vi "U6 Two 32-bit Frequency Measurements.vi"() -> ()   [LabVIEW 2021]
panel:
  in  "DeviceType":u16(ring)=1 items=["LJ_dtU3", "LJ_dtU6", "LJ_dtUE9"]
  out "Counter1 Diff (FIO3)":u32
  out "Frequency (FIO1)":dbl format="%.2f"
  out "Period (FIO1)":dbl format="%.6f"
  out "Iteration":i32
  out "Frequency (FIO0)":dbl format="%.2f"
  out "Period (FIO0)":dbl format="%.6f"
  in  "error in":errorcluster
  in  "ConnectionType":u16(ring) items=["LJ_ctUSB", "LJ_ctETHERNET"]
  in  "Address":string="1"
  in  "FirstFound":bool=TRUE
  in  "stop":bool
  out "Counter0 Diff (FIO2)":u32
  out "error out":errorcluster
  out "Error Message":string
  # "Each iteration, this VI measures the frequency on FIO0 and FIO1 using timer mode 2 (32-bit\nperiod measurement).  Also reads the count on FIO2 and FIO3 and\ndisplays the difference from the previous iteration, with the idea that the same signal can\nbe connected to FIO0 and FIO2 (and to FIO1 and FIO3) for comparison of period timing\nversus pulse counting."
  # "seconds"
  # "seconds"
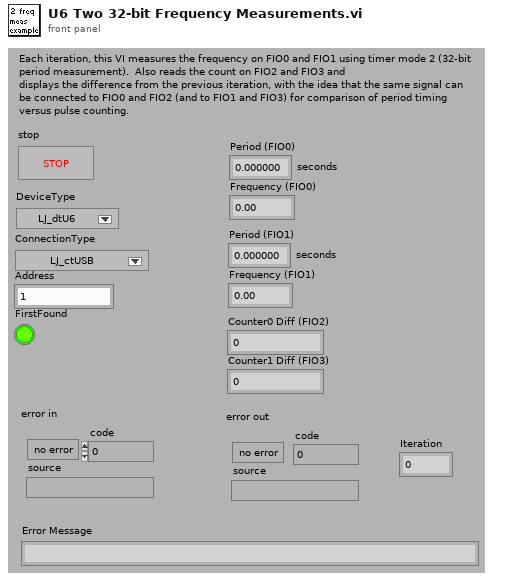
[diagram p1: front panel]
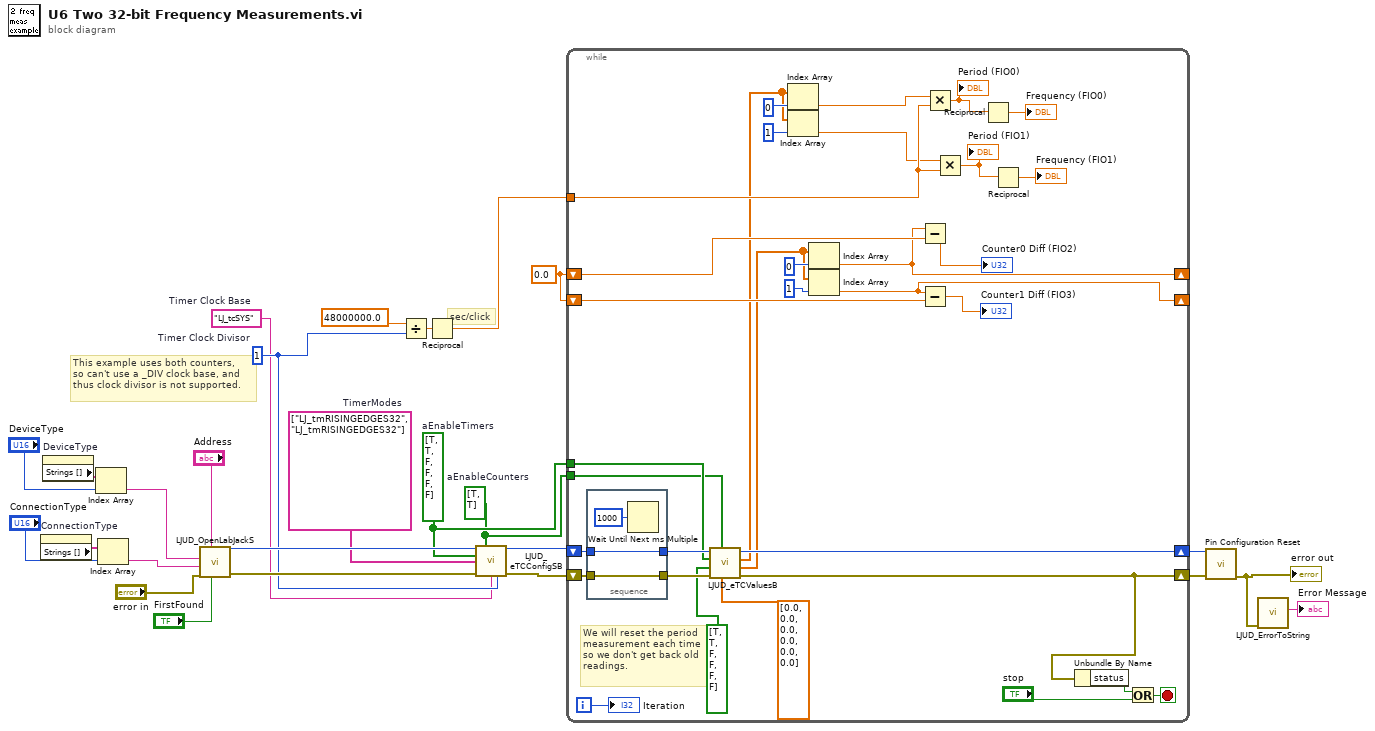
[diagram p0: block diagram]
diagram:
  w4 = bool[] [TRUE, TRUE]  # aEnableCounters
  w5 = bool[] [TRUE, TRUE, FALSE, FALSE, FALSE, FALSE]  # aEnableTimers
  w7 = 1  # Timer Clock Divisor
  w6 = "LJ_tcSYS"  # Timer Clock Base
  w8 = string[] ["LJ_tmRISINGEDGES32", "LJ_tmRISINGEDGES32"]  # TimerModes
  w19 = 0.0 ("TimerClockConfig")
  # "This example uses both counters,\nso can't use a _DIV clock base, and\nthus clock divisor is not supported."
  # "sec/click"
  n1 = property on="ConnectionType" class="Ring (strict)"() -> ("Strings []"=w17:string[])  [unwired: 2 in, 2 out]
  n2 = property on="DeviceType" class="Ring (strict)"() -> ("Strings []"=w18:string[])  [unwired: 2 in, 2 out]
  n3 = Index Array(array=w18, index="DeviceType") -> (element=w13:string)
  n4 = Index Array(array=w17, index="ConnectionType") -> (element=w14:string)
  n5 = call "LJUD_OpenLabJackS.vi"("FirstFound"="FirstFound", "Address"="Address", "error in"="error in", "ConnectionType"=w14, "DeviceType"=w13) -> ("error out"=w9:errorcluster, "Handle"=w10:i32)  [unwired: 4 in, 1 out]
  n6 = Divide(x=48000000.0, y=w7) -> (x/y=w21:dbl)
  n7 = Reciprocal(x=w21) -> (1/x=w20:dbl)
  n8 = call "LJUD_eTCConfigSB.vi"("Handle In"=w10, "aEnableCounters"=w4, "aEnableTimers"=w5, "aTimerModes"=w8, "error in"=w9, "TimerClockBase"=w6, "TimerClockDivisor"=w7) -> ("Handle Out"=w12:i32, "error out"=w11:errorcluster)  [unwired: 7 in]
  n9 = while {
    tunnel: w4 -> [w27]
    tunnel: w5 -> [w38]
    shift-left: w19 -> [w44]
    shift-right: [w28] -> _
    shift-left: w19 -> [w50]
    shift-right: [w29] -> _
    tunnel: w20 -> [w45]
    shift-left: w11 -> [w58]
    shift-right: [w41] -> w2
    shift-left: w12 -> [w59]
    shift-right: [w42] -> w3
    i -> [w48]
    stop <- w55 stop-if-true
    # "We will reset the period\nmeasurement each time\nso we don't get back old\nreadings."
    n10 = stacked-sequence {
      tunnel: [w61] -> w57
      tunnel: [w60] -> w56
      tunnel: w59 -> [w61]
      tunnel: w58 -> [w60]
      frame #0 {
        n11 = Wait Until Next ms Multiple(millisecond multiple=u32 1000) -> ()  [unwired: 1 out]
      }
    }
    n12 = call "LJUD_eTCValuesB.vi"("aTimerValues Write"=dbl[] [0.0, 0.0, 0.0, 0.0, 0.0, 0.0] ("TimerValues"), "aReadCounters"=w27, "error in"=w56, "aUpdateResetTimers"=bool[] [TRUE, TRUE, FALSE, FALSE, FALSE, FALSE] ("UpdateReset Timers"), "aReadTimers"=w38, "Handle In"=w57) -> ("error out"=w41:errorcluster, "aCounterValues"=w30:dbl[], "aTimerValues Read"=w35:dbl[], "Handle Out"=w42:i32)  [unwired: 2 in]
    n13 = Index Array(array=w35, index=0 ("Index")) -> (element=w34:dbl)
    n14 = Index Array(array=w35, index=1 ("Index")) -> (element=w33:dbl)
    n15 = Index Array(array=w30, index=0 ("Index")) -> (element=w29:dbl)
    n16 = Index Array(array=w30, index=1 ("Index")) -> (element=w28:dbl)
    n17 = Subtract(x=w29, y=w50) -> (x-y=→"Counter0 Diff (FIO2)":dbl)
    n18 = Subtract(x=w28, y=w44) -> (x-y=→"Counter1 Diff (FIO3)":dbl)
    n19 = Multiply(x=w34, y=w45) -> (x*y=w52:dbl)
    "Period (FIO0)" <- w52
    n20 = Multiply(x=w33, y=w45) -> (x*y=w47:dbl)
    "Period (FIO1)" <- w47
    n21 = Reciprocal(x=w52) -> (1/x=→"Frequency (FIO0)":dbl)
    n22 = Reciprocal(x=w47) -> (1/x=→"Frequency (FIO1)":dbl)
    n23 = Unbundle By Name(w41) -> ("status"=w54:bool)
    n24 = Or(x=w54, y="stop") -> (x .or. y?=w55:bool)
    "Iteration" <- w48
  }
  n25 = call "Pin Configuration Reset.vi"("error in"=w2, "Handle In"=w3) -> ("error out"=w1:errorcluster)  [unwired: 8 in, 1 out]
  "error out" <- w1
  n26 = call "LJUD_ErrorToString.vi"("error in"=w1) -> ("String"=→"Error Message":string)  [unwired: 10 in]
